vi "getDescriptor.vi"(8 "error in (no error)":errorcluster, 11 "ISignal in":refnum<class "ISignal.lvclass">) -> (0 "error out":errorcluster, 2 "DataDescriptor out":refnum<class "IDataDescriptor.lvclass">, 3 "ISignal out":refnum<class "ISignal.lvclass">)   [LabVIEW 2022 SP3, in "openDAQ.lvlib" / "IBaseObject.lvlib" / "IPropertyObject.lvlib" / "IComponent.lvlib" / "ISignal.lvlib" / "ISignal.lvclass"]
uses:
  <instrlib>/openDAQ/Public/Classes/ISignal/ISignal.lvclass
  <instrlib>/openDAQ/Public/Classes/ISignal/ISignal.lvclass/ISignal.ctl
  <instrlib>/openDAQ/Public/Classes/IDataDescriptor/IDataDescriptor.lvclass
  <instrlib>/openDAQ/Binaries/Windows/x86/copendaq32.dll
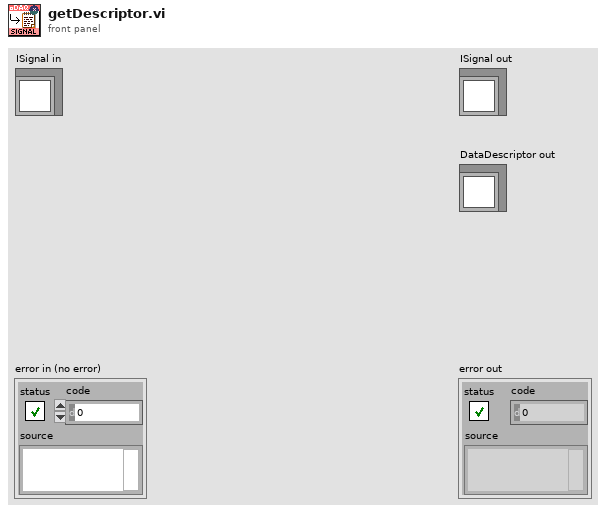
[diagram p1: front panel]
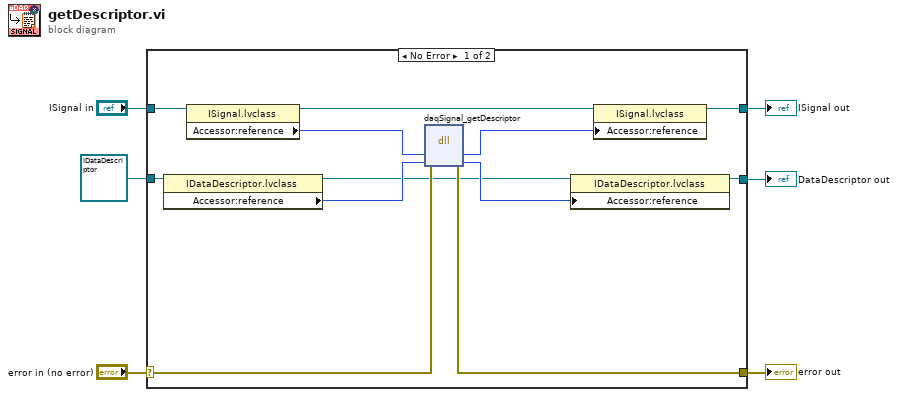
[diagram p0: block diagram]
diagram:
  n1 = case shown="No Error" "error in (no error)" {
    selector: "error in (no error)" -> [w16 w21]
    tunnel: [w15 w21] -> w5
    tunnel: [w10 w20] -> w3
    tunnel: "ISignal in" -> [w17 w20]
    tunnel: refnum<class "IDataDescriptor.lvclass"> refnum ("DataDescriptor in") -> [w14 w19]
    tunnel: [w8 w19] -> w1
    frame No Error {
      n2 = property class="IDataDescriptor.lvclass"(reference=w14) -> (reference out=w9:refnum<class "IDataDescriptor.lvclass">, "Accessor:reference"=w12:i64)  [unwired: 1 in, 1 out]
      n3 = property class="ISignal.lvclass"(reference=w17) -> (reference out=w11:refnum<class "ISignal.lvclass">, "Accessor:reference"=w13:i64)  [unwired: 1 in, 1 out]
      n4 = dll-call lib="C:/Program Files (x86)/National Instruments/LabVIEW 2022/instr.lib/openDAQ/Binaries/Windows/x86/copendaq*.*" fn="daqSignal_getDescriptor"(error in=w16, "signal"=w13, "descriptor"=w12) -> (error out=w15:errorcluster, "signal"=w7:i64, "descriptor"=w18:i64)  [unwired: 3 in, 1 out]
      n5 = property class="IDataDescriptor.lvclass"(reference=w9, "Accessor:reference"=w18) -> (reference out=w8:refnum<class "IDataDescriptor.lvclass">)  [unwired: 1 in, 1 out]
      n6 = property class="ISignal.lvclass"(reference=w11, "Accessor:reference"=w7) -> (reference out=w10:refnum<class "ISignal.lvclass">)  [unwired: 1 in, 1 out]
    }
    frame Error {
    }
  }
  "error out" <- w5
  "ISignal out" <- w3
  "DataDescriptor out" <- w1
